vi "Read Self Actor Attributes.vi"(7 "Actor in":refnum<data-value>) -> (2 "Self Actor Attributes":refnum<data-value>)   [LabVIEW 2020, in "jettl.lvlib"]
uses:
  jettl.lvlib
  Actor/Actor.lvclass
  Msg/Msg.lvclass
  Msgs.ctl
  Transport/Transport.lvclass
  Unified Layer.ctl
  Actor Attributes.ctl
  Layer.ctl
  Refs/Refs.lvclass
  Actor.ctl
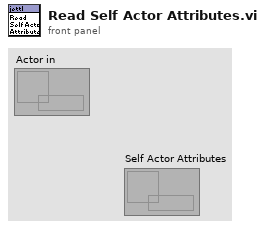
[diagram p1: front panel]
types:
  T1 = typedef "jettl.lvlib/Actor.ctl" = cluster{"Layer":T2, "Actor":refnum<class "Actor.lvclass">, "Refs":refnum<class "Refs.lvclass">}
  T2 = typedef "jettl.lvlib/Layer.ctl" = cluster{"Msgs":T3, "Leaf":bool, "Index":i32}
  T3 = typedef "jettl.lvlib/Msgs.ctl" = set{refnum<class "Msg.lvclass">}
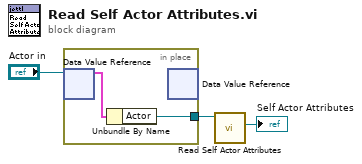
[diagram p0: block diagram]
diagram:
  n1 = in-place {
    in-place-border: [w4] -> w1
    n2 = in-place-dvr #1("Actor in") -> (w5:T1)  [unwired: 1 out]
    n3 = Unbundle By Name(w5) -> ("Actor"=w4:refnum<class "Actor.lvclass">)
    n4 = in-place-dvr #1() -> ()  [unwired: 1 in, 2 out]
  }
  n5 = call-dynamic "Read Self Actor Attributes.vi"("Actor in"=w1) -> ("Self Actor Attributes"=→"Self Actor Attributes":refnum<data-value>)  [unwired: 10 in]
